vi "ComboBox - Convert String To Enum.vi"(8 "Error In":errorcluster, 11 "Display Order (ComboBox string)":string) -> (0 "Error Out":errorcluster, 3 "Display Order (enum)":T1)   [LabVIEW 2023, in "Error Manager.lvlib"]
doc: "Blank VI with error handling."
uses:
  Error Manager.lvlib
  Display Order (enum).ctl
panel:
  # "Input\nInputs to the VI"
  # "Development\nControls or indicators that are useful for development or testing, but which are not outputs of the VI."
  # "Output\nOutputs of the VI"
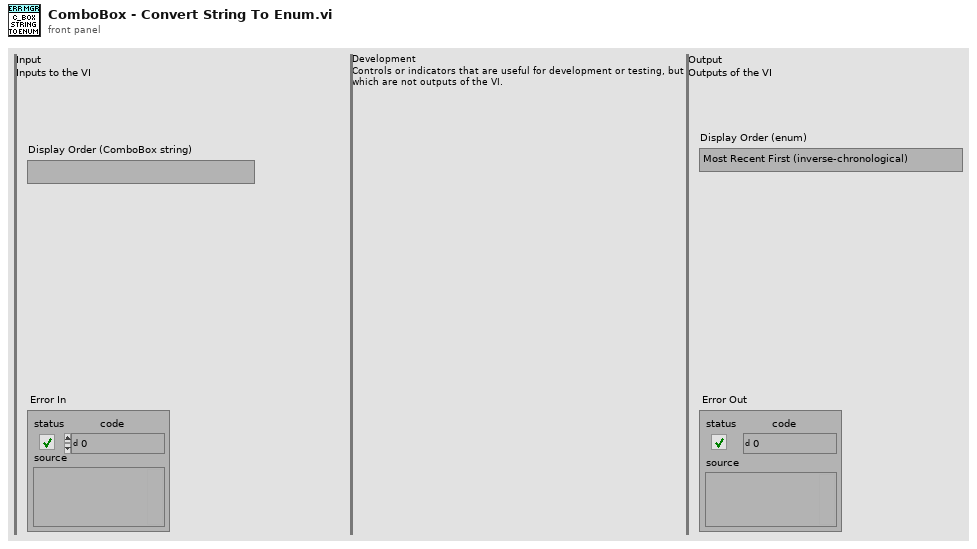
[diagram p1: front panel]
types:
  T1 = typedef "Error Manager.lvlib/Display Order (enum).ctl" = enum16{"Most Recent First (inverse-chronological)", "Oldest First (chronological)"}
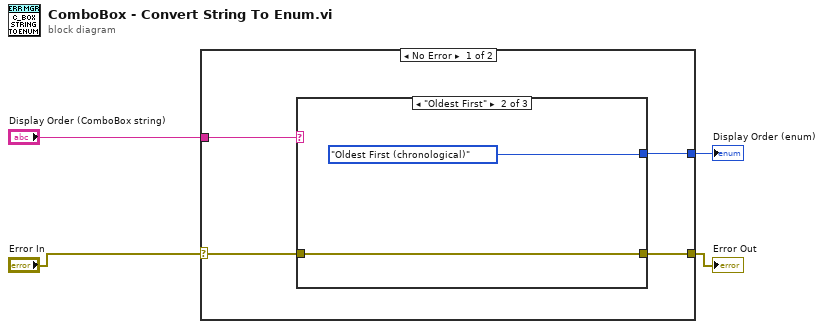
[diagram p0: block diagram]
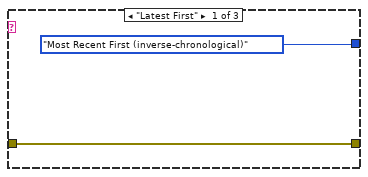
[diagram p2: hidden frame]
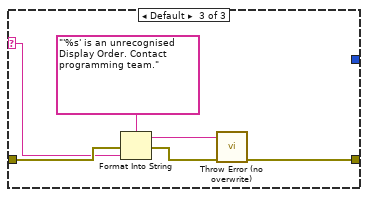
[diagram p3: hidden frame]
diagram:
  n1 = case shown="No Error" "Error In" {
    selector: "Error In" -> [w8 w19]
    tunnel: [w7 w19] -> w3
    tunnel: "Display Order (ComboBox string)" -> [w6 _]
    tunnel: [w5 _] -> w1
    frame No Error {
      n2 = case shown="\"Oldest First\"" w6 {
        selector: w6 -> [_ _ w15]
        tunnel: w8 -> [w9 w12 w16]
        tunnel: [w9 w12 w18] -> w7
        tunnel: [Display_Order_(enum)."Most Recent First (inverse-chronological)" ("Display Order (enum)") Display_Order_(enum)."Oldest First (chronological)" ("Display Order (enum)") _] -> w5
        frame "Latest First" {
        }
        frame "Oldest First" {
        }
        frame Default {
          n3 = Format Into String(format string="'%s' is an unrecognised Display Order. Contact programming team.", error in=w16, w15) -> (resulting string=w14:string, error out=w17:errorcluster)  [unwired: 1 in]
          n4 = call "Throw Error (no overwrite).vi"("error in"=w17, "Error Message (\"\")"=w14) -> ("error out"=w18:errorcluster)  [unwired: 9 in]
        }
      }
    }
    frame Error {
    }
  }
  "Error Out" <- w3
  "Display Order (enum)" <- w1
